vi "Scanner_main_16_3D_2chan.vi"() -> ()   [LabVIEW 2016]
uses:
  <vilib>/DAQmx/write.llb/DAQmx Write (Digital Bool 1Line 1Point).vi
  <vilib>/DAQmx/read.llb/DAQmx Read (Analog 1D DBL 1Chan NSamp).vi
  <vilib>/DAQmx/write.llb/DAQmx Write (Analog 1D Wfm NChan NSamp).vi
  <vilib>/DAQmx/read.llb/DAQmx Read (Counter 1D DBL 1Chan NSamp).vi
  <vilib>/DAQmx/create/channels.llb/DAQmx Create Channel (DO-Digital Output).vi
  <vilib>/DAQmx/miscellaneous.llb/DAQmx Fill In Error Info.vi
  <vilib>/DAQmx/create/channels.llb/DAQmx Create Channel (AI-Voltage-Basic).vi
  <vilib>/DAQmx/configure/timing.llb/DAQmx Timing (Sample Clock).vi
  <vilib>/DAQmx/configure/trigger.llb/DAQmx Start Trigger (Digital Edge).vi
  <vilib>/DAQmx/create/channels.llb/DAQmx Create Channel (CI-Count Edges).vi
  <vilib>/DAQmx/create/channels.llb/DAQmx Create Channel (AO-Voltage-Basic).vi
  <resource>/objmgr/daqmx.rc
panel:
  out "saved .ids":bool
  out "Reflection":dbl[][](graph)
  out "End_of_Stack":bool
  out "refnum out":refnum<file>
  out "Numeric":i32
  out "path to .ids 2":path
  out "x = y?":bool
  out "Z positions":dbl[](array[numeric])
  out "piezo_step":bool
  out "step (um)":dbl
  out "Z position":dbl format="%.6f"
  out "Z step (um)":dbl
  out "System no.":i32=1
  out "Conn. Axes":string[](array[string])
  out "Piezo status":bool
  out "path to .ids":path
  out "saved .ics":bool
  in  "folder":path=path "C:/Users/Sergey/Scan"
  in  "filename":string="PSF2"
  in  "Range Z:":dbl=10.0
  in  "Slices Z:":i32=50
  out "Scan_pix":i32
  out "Frame:":i32
  out "length of scan":i32
  in  "OK Button":bool
  in  "delta_p":i32=-24
  out "Current Line:":i32
  in  "Y":dbl
  in  "offset X:":dbl
  in  "stop":bool
  in  "Save":bool=TRUE
  in  "Range:":dbl=45.0
  in  "Pixels:":i32=650
  in  "Dwell:":dbl=5e-05 format="%#_6p"
  out "Fluorescence":i32[][](graph) caption="Intensity Graph"
  # "Scan:"
  # "Nyquist 0.073um"
  # "Nyquist 0.23um"
  # "Z-position:"
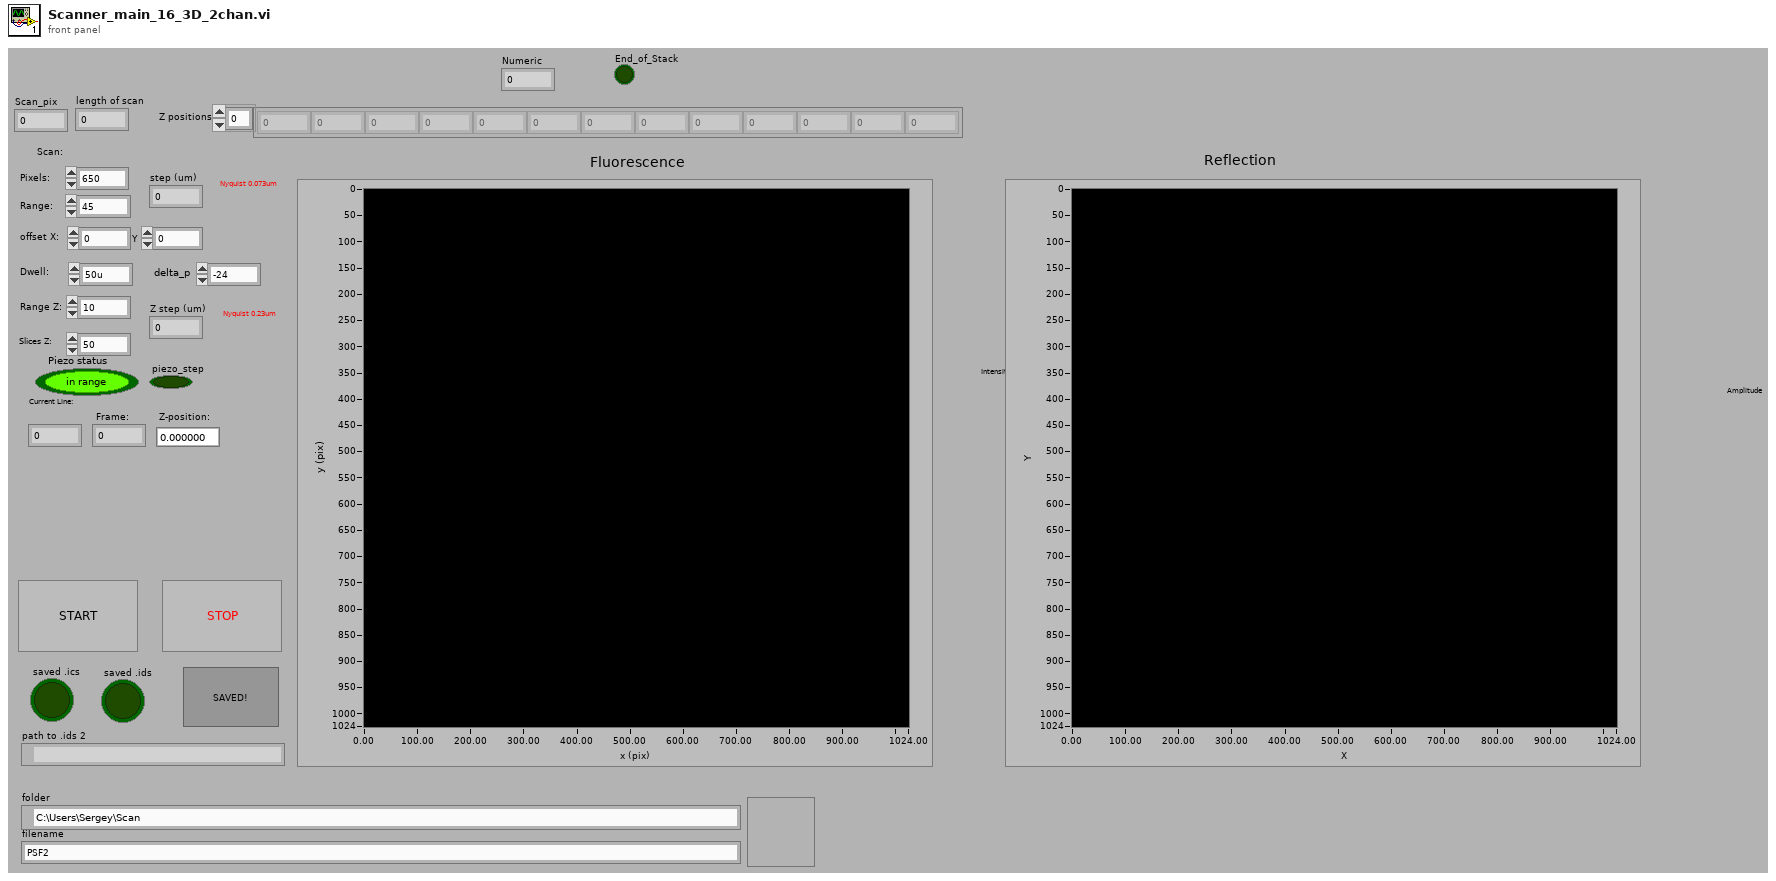
[diagram p1: front panel]
types:
  T1 = enum16{"open", "replace", "create", "open or create", "replace or create", "replace or create with confirmation"}
  T2 = enum16{"big-endian, network order", "native, host order", "little-endian"}
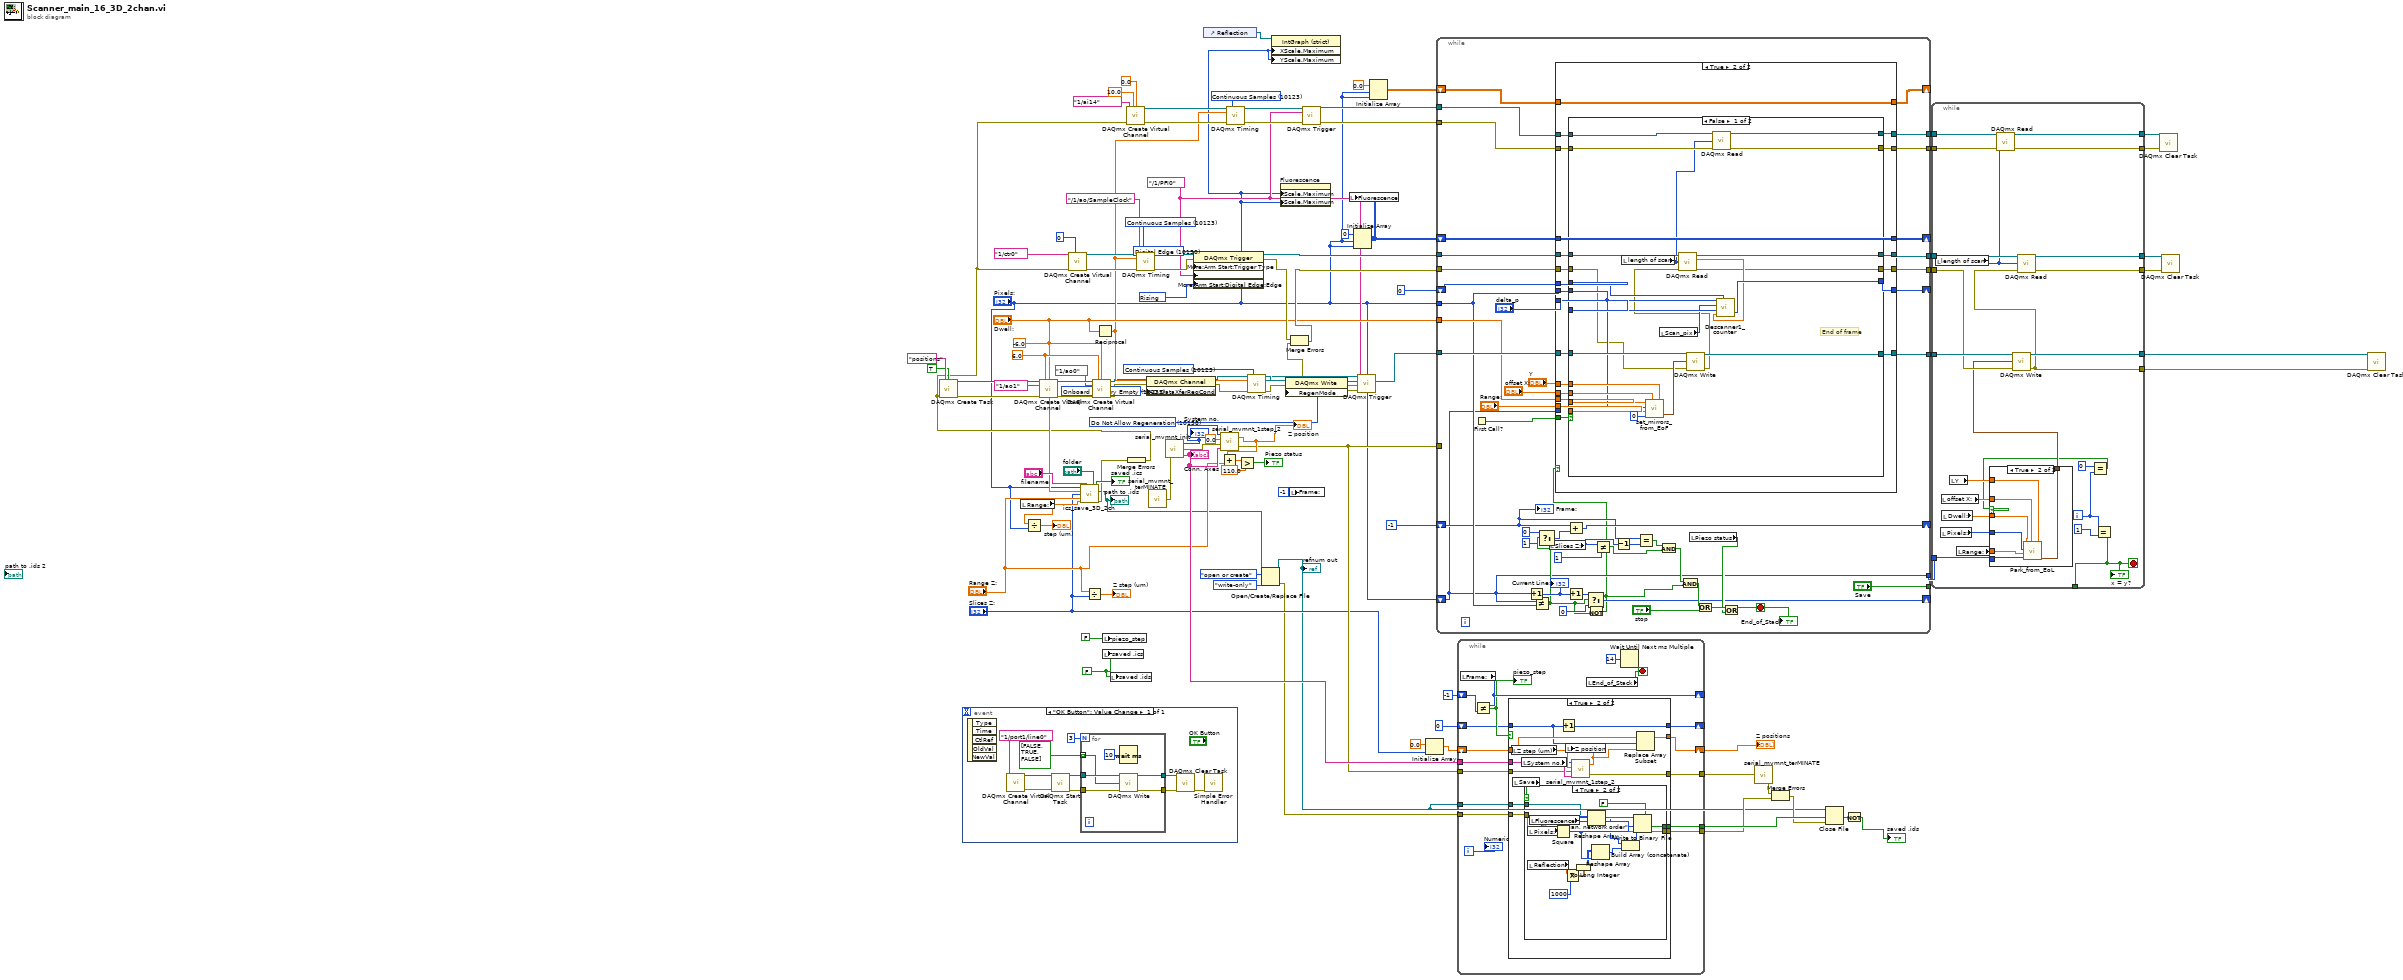
[diagram p0: block diagram]
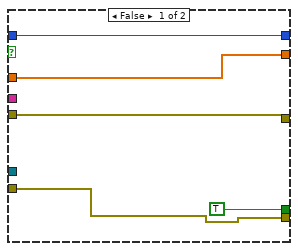
[diagram p2: hidden frame]
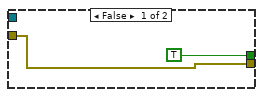
[diagram p3: hidden frame]
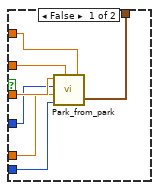
[diagram p4: hidden frame]
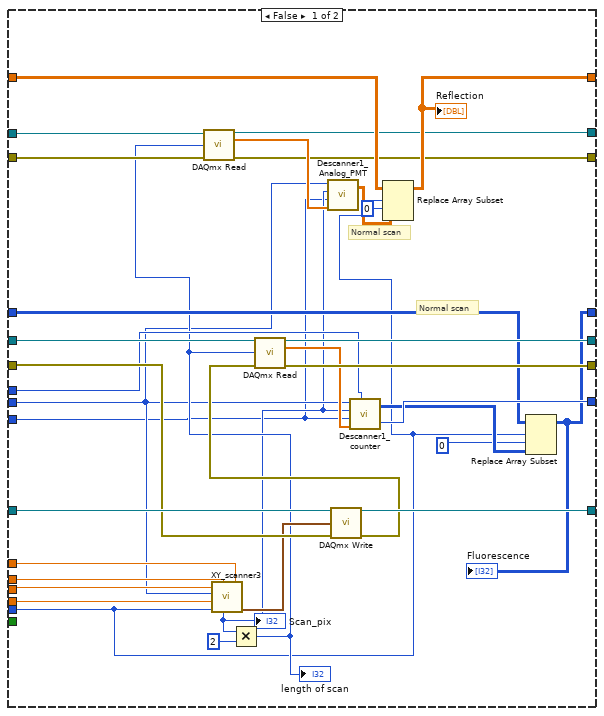
[diagram p5: hidden frame]
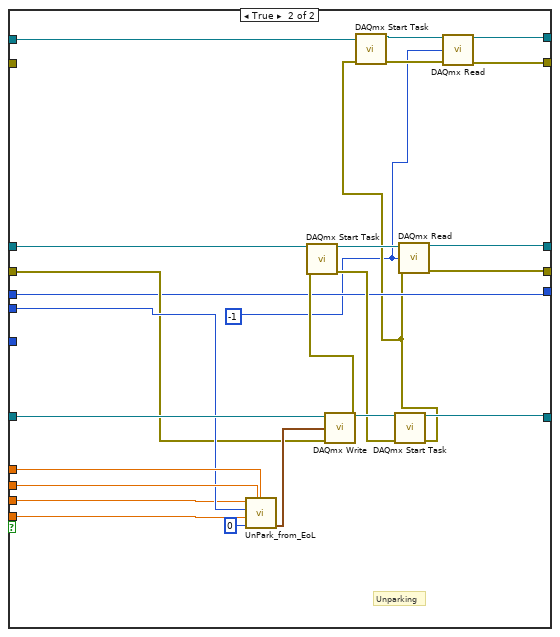
[diagram p6: hidden frame]
diagram:
  w5 = 10235 items=["Onboard Memory Empty"=10235, "Onboard Memory Half Full or Less"=10239, "Onboard Memory Less than Full"=10242] ("AO.DataXferReqCond")
  w30 = 10123 items=["Finite Samples"=10178, "Continuous Samples"=10123] ("sample mode")
  w3 = FALSE ("saved")
  w85 = 10280 items=["Rising"=10280, "Falling"=10171] ("ArmStart.DigEdge.Edge")
  w20 = tag "/1/PFI0" ("ArmStart.DigEdge.Src")
  w86 = 10150 items=["Digital Edge"=10150, "None"=10230] ("ArmStart.TrigType")
  w97 = 10158 items=["Allow Regeneration"=10097, "Do Not Allow Regeneration"=10158] ("RegenMode")
  w101 = 6.0 ("maximum value")
  w100 = -6.0 ("minimum value")
  w105 = 10123 items=["Finite Samples"=10178, "Continuous Samples"=10123] ("sample mode")
  w108 = 10123 items=["Finite Samples"=10178, "Continuous Samples"=10123] ("sample mode")
  n1 = event shown="[0] \"OK Button\": Value Change" {
    selector: _ -> [_]
    dyn-events: _ -> [_]
    timeout: _ -> [_]
    event "OK Button": Value Change {
      n2 = event-data() -> ()  [unwired: 6 out]
      n3 = call-poly <vilib>:"DAQmx Create Virtual Channel.vi"("lines"=tag "1/port1/line0" ("Software Trigger Line")) -> ("task out"=w117:refnum<k21>, "error out"=w116:errorcluster)  [unwired: 4 in, 9 out]
      n4 = call <vilib>:"DAQmx Start Task.vi"("task/channels in"=w117, "error in"=w116) -> ("task out"=w115:refnum<k21>, "error out"=w114:errorcluster)  [unwired: 12 out]
      n5 = for {
        N: 3 -> [_]
        tunnel: w115 -> [w123]
        tunnel: w114 -> [w122]
        tunnel: bool[] [FALSE, TRUE, FALSE] -> [w121] mode=indexing
        tunnel: [w120] -> w111
        tunnel: [w119] -> w110
        n6 = Wait (ms)(milliseconds to wait=u32 10) -> ()  [unwired: 1 out]
        n7 = call-poly <vilib>:"DAQmx Write.vi"("task/channels in"=w123, "data"=w121, "error in"=w122) -> ("task out"=w119:refnum<k21>, "error out"=w120:errorcluster)  [unwired: 1 in, 10 out]
      }
      n8 = call <vilib>:"DAQmx Clear Task.vi"("task in"=w110, "error in"=w111) -> ("error out"=w112:errorcluster)  [unwired: 13 out]
      n9 = call <vilib>:"Simple Error Handler.vi"("error in (no error)"=w112) -> ()  [unwired: 1 in, 8 out]
    }
  }
  n10 = local read "Range:"() -> (w44:dbl)
  n11 = Divide(x=w44, y="Pixels:") -> (x/y=→"step (um)":dbl)
  n12 = call "ics_save_3D_2ch.vi"("pixels"="Pixels:", "filename"="filename", "folder"="folder", "Dwell"="Dwell:", "slices Z"="Slices Z:", "Range Z"="Range Z:", "Range"=w44) -> ("saved"=→"saved .ics":bool, "path to .ids"=w40:path, "error out"=w61:errorcluster)  [unwired: 6 in]
  "path to .ids" <- w40
  n13 = Divide(x="Range Z:", y="Slices Z:") -> (x/y=→"Z step (um)":dbl)
  n14 = Reciprocal(x="Dwell:") -> (1/x=w21:dbl)
  n15 = local write "piezo_step"(FALSE ("x != y?")) -> ()
  n16 = local write "saved .ics"(w3) -> ()
  n17 = local write "saved .ids"(w3) -> ()
  n18 = Merge Errors(w61) -> (w11:errorcluster)
  n19 = call <vilib>:"DAQmx Create Task.vi"("new task name"="positions", "auto cleanup"=TRUE, "error in"=w11) -> ("task out"=w94:refnum<k21>, "error out"=w91:errorcluster)  [unwired: 11 in]
  n20 = call-poly <vilib>:"DAQmx Create Virtual Channel.vi"("task in"=w94, "maximum value"=w101, "minimum value"=w100, "physical channels"=tag "1/ao1", "error in"=w91) -> ("task out"=w104:refnum<k21>, "error out"=w103:errorcluster)  [unwired: 9 in]
  n21 = call-poly <vilib>:"DAQmx Create Virtual Channel.vi"("initial count"=u32 0, "counter"=tag "1/ctr0", "error in"=w11) -> ("task out"=w95:refnum<k21>, "error out"=w107:errorcluster)  [unwired: 11 in]
  n22 = call-poly <vilib>:"DAQmx Create Virtual Channel.vi"("task in"=w104, "maximum value"=w101, "minimum value"=w100, "physical channels"=tag "1/ao0" ("physical channels 2"), "error in"=w103) -> ("task out"=w9:refnum<k21>, "error out"=w7:errorcluster)  [unwired: 9 in]
  n23 = call-poly <vilib>:"DAQmx Create Virtual Channel.vi"("maximum value"=10.0, "minimum value"=0.0, "physical channels"=tag "1/ai14", "error in"=w11) -> ("task out"=w26:refnum<k21>, "error out"=w25:errorcluster)  [unwired: 10 in]
  n24 = call-poly <vilib>:"DAQmx Timing.vi"("task/channels in"=w95, "sample mode"=w108, "rate"=w21, "source"=tag "/1/ao/SampleClock", "error in"=w107) -> ("task out"=w88:refnum<k21>, "error out"=w87:errorcluster)  [unwired: 9 in]
  n25 = property class="DAQmx Channel"(reference=w9, error in=w7, "AO.DataXferReqCond"=w5) -> (reference out=w8:refnum<k21>, error out=w6:errorcluster)
  n26 = call "serial_mvmnt_terMINATE.vi"() -> ("error out"=w55:errorcluster)  [unwired: 1 in]
  n27 = call "serial_mvmnt_init.vi"("error in"=w55) -> ("System no."=w59:i32, "error out"=w58:errorcluster, "Conn. Axes"=w54:string[])
  "Conn. Axes" <- w54
  "System no." <- w59
  n28 = property class="DAQmx Trigger"(reference=w88, error in=w87, "More:Arm Start:Trigger Type"=w86, "More:Arm Start:Digital Edge:Source"=w20, "More:Arm Start:Digital Edge:Edge"=w85) -> (reference out=w79:refnum<k21>, error out=w84:errorcluster)
  n29 = control-ref of="Reflection"() -> (w2:refnum<vi>)
  n30 = call "serial_mvmnt_1step_2.vi"("Conn. Axes"=w54, "error in"=w58, "Z step"=0.0, "System no."=w59) -> ("error out"=w53:errorcluster, "Position"=w56:dbl)
  "Z position" <- w56
  n31 = Add(x=w56, y="Range Z:") -> (x+y=w64:dbl)
  n32 = call-poly <vilib>:"DAQmx Timing.vi"("task/channels in"=w26, "sample mode"=w30, "rate"=w21, "error in"=w25) -> ("task out"=w24:refnum<k21>, "error out"=w23:errorcluster)  [unwired: 10 in]
  n33 = Greater?(x=w64, y=110.0) -> (0:→"Piezo status":bool)
  n34 = call-poly <vilib>:"DAQmx Timing.vi"("task/channels in"=w8, "sample mode"=w105, "rate"=w21, "error in"=w6) -> ("task out"=w99:refnum<k21>, "error out"=w10:errorcluster)  [unwired: 10 in]
  n35 = Open/Create/Replace File(file path (use dialog)=w40, operation (0:open)=T1."open or create", access (0:read/write)=enum16{"read/write", "read-only", "write-only"}."write-only") -> (refnum out=w33:refnum<file>, error out=w38:errorcluster)  [unwired: 3 in, 1 out]
  "refnum out" <- w33
  n36 = property on="Property Node" class="IntGraph (strict)"(reference=w2, "XScale.Maximum"="Pixels:", "YScale.Maximum"="Pixels:") -> ()  [unwired: 1 in, 2 out]
  n37 = property on="Fluorescence" class="IntGraph (strict)"("XScale.Maximum"="Pixels:", "YScale.Maximum"="Pixels:") -> ()  [unwired: 2 in, 2 out]
  n38 = property class="DAQmx Write"(reference=w99, error in=w10, "RegenMode"=w97) -> (reference out=w83:refnum<k21>, error out=w82:errorcluster)
  n39 = local write "Frame:"(-1 ("Frame:")) -> ()
  n40 = call-poly <vilib>:"DAQmx Trigger.vi"("task/channels in"=w24, "source"=w20, "error in"=w23) -> ("task out"=w19:refnum<k21>, "error out"=w18:errorcluster)  [unwired: 11 in]
  n41 = Initialize Array(0 ("element"), "Pixels:", "Pixels:") -> (w37:i32[][])
  n42 = local write "Fluorescence"(w37) -> ()
  n43 = call-poly <vilib>:"DAQmx Trigger.vi"("task/channels in"=w83, "source"=w20, "error in"=w82) -> ("task out"=w80:refnum<k21>, "error out"=w81:errorcluster)  [unwired: 11 in]
  n44 = Merge Errors(w84, w81) -> (w78:errorcluster)
  n45 = Initialize Array(0.0 ("element"), "Pixels:", "Pixels:") -> (w17:dbl[][])
  n46 = Initialize Array(0.0 ("element"), "Slices Z:") -> (w46:dbl[])
  n47 = while {
    tunnel: w80 -> [w162]
    tunnel: w79 -> [w158]
    tunnel: w78 -> [w157]
    tunnel: "Pixels:" -> [w151]
    tunnel: "Dwell:" -> [w153]
    shift-right: [w133] -> _
    shift-left: "Pixels:" -> [w134]
    tunnel: [w165] -> w75
    shift-right: [w159] -> _
    shift-left: w37 -> [w160]
    tunnel: ["Save"] -> _
    tunnel: [w164] -> w76
    tunnel: [w163] -> w77
    tunnel: [w134] -> w71
    shift-right: [w138] -> _
    shift-left: -1 ("t") -> [w135]
    shift-right: [w145] -> _
    shift-left: 0 ("t") -> [w146]
    tunnel: w53 -> [_]
    tunnel: w19 -> [w129]
    tunnel: w18 -> [w128]
    shift-right: [w127] -> _
    shift-left: w17 -> [w130]
    tunnel: [w126] -> w16
    tunnel: [w125] -> w15
    stop <- w131 stop-if-true
    n48 = First Call?() -> (First Call?: T/F=w152:bool)
    n49 = Increment(x=w134) -> (x+1=w168:i32)
    "Current Line:" <- w168
    n50 = Not Equal?(x=w134, y=w151) -> (x != y?=w149:bool)
    n51 = Select(t=0, s=w149, f=1) -> (s? t:f=w150:i32)
    n52 = local read "Slices Z:"() -> (w143:i32)
    n53 = Add(x=w135, y=w150) -> (x+y=w138:i32)
    n54 = Increment(x=w168) -> (x+1=w166:i32)
    n55 = Select(t=w166, s=w149, f=0) -> (s? t:f=w133:i32)
    n56 = Not(x=w149) -> (.not. x?=w132:bool)
    n57 = case shown="True" w132 {
      tunnel: [w202 w225] -> w164
      tunnel: w158 -> [w203 w226]
      tunnel: [w201 w222] -> w165
      tunnel: w157 -> [w194 w221]
      tunnel: [w204 w223] -> w163
      tunnel: w162 -> [w205 w224]
      tunnel: "delta_p" -> [w173 w212]
      tunnel: w151 -> [w175 w215]
      tunnel: w160 -> [w188 w211]
      tunnel: [w186 w211] -> w159
      tunnel: "Y" -> [w200 w220]
      tunnel: "offset X:" -> [w199 w219]
      tunnel: w153 -> [w198 w218]
      tunnel: "Range:" -> [w197 w217]
      tunnel: w134 -> [w172 _]
      tunnel: w152 -> [_ w216]
      tunnel: w146 -> [w192 w213]
      tunnel: [w191 w214] -> w145
      tunnel: w130 -> [w182 w206]
      tunnel: w129 -> [w181 w210]
      tunnel: w128 -> [w180 w209]
      tunnel: [w179 w206] -> w127
      tunnel: [w178 w208] -> w126
      tunnel: [w177 w207] -> w125
      frame False {
        # "Normal scan"
        # "Normal scan"
        n58 = call "XY_scanner3.vi"("offset Y"=w200, "offset X"=w199, "Line_start"=w172, "Range"=w197, "Pixels"=w175, "dwell"=w198) -> ("X and Y"=w193:waveform(dbl)[], "scanPix"=w174:i32)  [unwired: 2 out]
        "Scan_pix" <- w174
        n59 = Multiply(x=w174, y=2) -> (x*y=w176:i32)
        "length of scan" <- w176
        n60 = call-poly <vilib>:"DAQmx Read.vi"("task/channels in"=w181, "number of samples per channel"=w176, "error in"=w180) -> ("task out"=w178:refnum<k21>, "data"=w185:dbl[], "error out"=w177:errorcluster)  [unwired: 10 in]
        n61 = call "Descanner1_Analog_PMT.vi"("Pix"=w175, "scanPix"=w174, "delta_p"=w173, "Data"=w185) -> ("2Lines"=w183:dbl[][])  [unwired: 2 in]
        n62 = call-poly <vilib>:"DAQmx Write.vi"("task/channels in"=w205, "data"=w193, "error in"=w194) -> ("task out"=w204:refnum<k21>, "error out"=w195:errorcluster)  [unwired: 10 in, 1 out]
        n63 = call-poly <vilib>:"DAQmx Read.vi"("task/channels in"=w203, "number of samples per channel"=w176, "error in"=w195) -> ("task out"=w202:refnum<k21>, "data"=w190:dbl[], "error out"=w201:errorcluster)  [unwired: 10 in]
        n64 = call "Descanner1_counter.vi"("Pix"=w175, "scanPix"=w174, "delta_p"=w173, "Data"=w190, "last_count prev line"=w192) -> ("2Lines"=w189:i64[][], "last_count"=w191:i64)
        n65 = Replace Array Subset(array=w182, new element=w183, index (row)=w172, index (col)=0 ("disabled index (col)")) -> (w179:dbl[][])
        "Reflection" <- w179
        n66 = Replace Array Subset(array=w188, new element=w189, index (row)=w172, index (col)=0 ("disabled index (col)")) -> (w186:i32[][])
        "Fluorescence" <- w186
      }
      frame True {
        n67 = case shown="False" w216 {
          tunnel: w226 -> [w250 w264]
          tunnel: [w249 w259] -> w225
          tunnel: w224 -> [w248 w275]
          tunnel: [w247 w266] -> w223
          tunnel: [w232 w258] -> w222
          tunnel: w215 -> [w236 w272]
          tunnel: w221 -> [w233 w265]
          tunnel: w220 -> [w243 w274]
          tunnel: w219 -> [w242 w273]
          tunnel: w218 -> [w245 w271]
          tunnel: w217 -> [w241 w270]
          tunnel: [w239 w261] -> w214
          tunnel: w213 -> [w240 w261]
          tunnel: w212 -> [w237 _]
          tunnel: w210 -> [w231 w251]
          tunnel: w209 -> [w230 _]
          tunnel: [w228 w255] -> w208
          tunnel: [w227 w254] -> w207
          frame False {
            # "End of frame"
            n68 = local read "length of scan"() -> (w229:i32)
            n69 = call "set_mirrors_from_EoF.vi"("offset Y"=w243, "offset X"=w242, "Line_start"=0, "Range"=w241, "Pixels"=w236, "dwell"=w245) -> ("X and Y"=w244:waveform(dbl)[])  [unwired: 1 out]
            n70 = local read "Scan_pix"() -> (w235:i32)
            n71 = call-poly <vilib>:"DAQmx Write.vi"("task/channels in"=w248, "data"=w244, "error in"=w233) -> ("task out"=w247:refnum<k21>, "error out"=w234:errorcluster)  [unwired: 10 in, 1 out]
            n72 = call-poly <vilib>:"DAQmx Read.vi"("task/channels in"=w250, "number of samples per channel"=w229, "error in"=w234) -> ("task out"=w249:refnum<k21>, "data"=w238:dbl[], "error out"=w232:errorcluster)  [unwired: 10 in]
            n73 = call-poly <vilib>:"DAQmx Read.vi"("task/channels in"=w231, "number of samples per channel"=w229, "error in"=w230) -> ("task out"=w228:refnum<k21>, "error out"=w227:errorcluster)  [unwired: 10 in, 1 out]
            n74 = call "Descanner1_counter.vi"("Pix"=w236, "scanPix"=w235, "delta_p"=w237, "Data"=w238, "last_count prev line"=w240) -> ("last_count"=w239:i64)  [unwired: 1 out]
          }
          frame True {
            w252 = -1 ("number of samples per channel")
            # "Unparking"
            n75 = call "UnPark_from_EoL.vi"("offset Y"=w274, "offset X"=w273, "Line_start"=0, "Range"=w270, "Pixels"=w272, "dwell"=w271) -> ("X and Y"=w268:waveform(dbl)[])  [unwired: 2 out]
            n76 = call-poly <vilib>:"DAQmx Write.vi"("task/channels in"=w275, "data"=w268, "error in"=w265) -> ("task out"=w267:refnum<k21>, "error out"=w263:errorcluster)  [unwired: 10 in, 1 out]
            n77 = call <vilib>:"DAQmx Start Task.vi"("task/channels in"=w264, "error in"=w263) -> ("task out"=w260:refnum<k21>, "error out"=w262:errorcluster)  [unwired: 12 in]
            n78 = call <vilib>:"DAQmx Start Task.vi"("task/channels in"=w267, "error in"=w262) -> ("task out"=w266:refnum<k21>, "error out"=w253:errorcluster)  [unwired: 12 in]
            n79 = call <vilib>:"DAQmx Start Task.vi"("task/channels in"=w251, "error in"=w253) -> ("task out"=w257:refnum<k21>, "error out"=w256:errorcluster)  [unwired: 12 in]
            n80 = call-poly <vilib>:"DAQmx Read.vi"("task/channels in"=w260, "number of samples per channel"=w252, "error in"=w253) -> ("task out"=w259:refnum<k21>, "error out"=w258:errorcluster)  [unwired: 10 in, 1 out]
            n81 = call-poly <vilib>:"DAQmx Read.vi"("task/channels in"=w257, "number of samples per channel"=w252, "error in"=w256) -> ("task out"=w255:refnum<k21>, "error out"=w254:errorcluster)  [unwired: 10 in, 1 out]
          }
        }
      }
    }
    n82 = Not Equal?(x=w143, y=1) -> (x != y?=w140:bool)
    n83 = Decrement(x=w143) -> (x-1=w142:i32)
    n84 = Equal?(x=w135, y=w142) -> (x = y?=w141:bool)
    n85 = And(x=w141, y=w140) -> (x .and. y?=w139:bool)
    n86 = And(x=w139, y=w132) -> (x .and. y?=w169:bool)
    n87 = local read "Piezo status"() -> (w136:bool)
    n88 = Or(x=w169, y="stop") -> (x .or. y?=w137:bool)
    n89 = Or(x=w137, y=w136) -> (x .or. y?=w131:bool)
    "End_of_Stack" <- w131
    "Frame:" <- w135
  }
  n90 = while {
    tunnel: w54 -> [w292]
    tunnel: w53 -> [w291]
    shift-right: [w290] -> _
    shift-left: -1 ("Frame") -> [w289]
    tunnel: [w288] -> w51
    shift-right: [w285] -> _
    shift-left: 0 ("Frame") -> [w286]
    shift-right: [w283] -> w32
    shift-left: w46 -> [w284]
    tunnel: [w281] -> w39
    tunnel: w38 -> [w279]
    tunnel: [w278] -> w35
    tunnel: w33 -> [w276]
    i -> [w280]
    stop <- w277 stop-if-true
    n91 = local read "Frame:"() -> (w290:i32)
    n92 = Not Equal?(x=w290, y=w289) -> (x != y?=w287:bool)
    "piezo_step" <- w287
    n93 = case shown="True" w287 {
      tunnel: w292 -> [_ w310]
      tunnel: w291 -> [w297 w309]
      tunnel: [w297 w308] -> w288
      tunnel: w286 -> [w296 w303]
      tunnel: [w296 w304] -> w285
      tunnel: w284 -> [w295 w307]
      tunnel: [w295 w306] -> w283
      tunnel: [TRUE ("cancelled") w301] -> w281
      tunnel: w279 -> [w293 w300]
      tunnel: [w293 w299] -> w278
      tunnel: w276 -> [_ w298]
      frame False {
      }
      frame True {
        n94 = local read "Z step (um)"() -> (w312:dbl)
        n95 = local read "Save"() -> (w302:bool)
        n96 = local read "System no."() -> (w311:i32)
        n97 = case shown="True" w302 {
          tunnel: [TRUE ("cancelled") w327] -> w301
          tunnel: w300 -> [w313 w326]
          tunnel: [w313 w325] -> w299
          tunnel: w298 -> [_ w324]
          frame False {
          }
          frame True {
            n98 = local read "Pixels:"() -> (w329:i32)
            n99 = local read "Reflection"() -> (w322:dbl[][])
            n100 = local read "Fluorescence"() -> (w328:i32[][])
            n101 = Square(x=w329) -> (x^2=w323:i32)
            n102 = Multiply(x=w322, y=1000) -> (x*y=w316:dbl[][])
            n103 = To Long Integer(number=w316) -> (32bit integer=w315:i32[][])
            n104 = Reshape Array(w328, w323) -> (w320:i32[])
            n105 = Reshape Array(w315, w323) -> (w319:i32[])
            n106 = Build Array (concatenate)(w320, w319) -> (w318:i32[])
            n107 = Write to Binary File(file (use dialog)=w324, data=w318, error in=w326, 5:FALSE ("prepend array or string size? (T)"), 9:T2."big-endian, network order" ("byte order (0:big-endian, network order)")) -> (cancelled=w327:bool, error out=w325:errorcluster)  [unwired: 1 in, 1 out]
          }
        }
        n108 = Increment(x=w303) -> (x+1=w304:i32)
        n109 = call "serial_mvmnt_1step_2.vi"("Conn. Axes"=w310, "error in"=w309, "Z step"=w312, "System no."=w311) -> ("error out"=w308:errorcluster, "Position"=w305:dbl)
        n110 = local write "Z position"(w305) -> ()
        n111 = Replace Array Subset(array=w307, new element=w305, index=w303) -> (w306:dbl[])
      }
    }
    n112 = local read "End_of_Stack"() -> (w277:bool)
    n113 = Wait Until Next ms Multiple(millisecond multiple=u32 14 ("milliseconds to wait")) -> ()  [unwired: 1 out]
    "Numeric" <- w280
  }
  "Z positions" <- w32
  n114 = call "serial_mvmnt_terMINATE.vi"("error in"=w51) -> ("error out"=w36:errorcluster)
  n115 = Merge Errors(w36, w35) -> (w34:errorcluster)
  n116 = Close File(refnum=w33, error in=w34) -> ()  [unwired: 2 out]
  n117 = Not(x=w39) -> (.not. x?=→"saved .ids":bool)
  n118 = while {
    tunnel: w77 -> [w354]
    tunnel: w71 -> [w353]
    tunnel: w76 -> [w352]
    tunnel: w75 -> [w351]
    tunnel: [w350] -> w73
    tunnel: [w349] -> w14
    tunnel: [w343] -> w74
    tunnel: [w337] -> w72
    tunnel: [w336] -> _
    tunnel: w16 -> [w335]
    tunnel: w15 -> [w334]
    tunnel: [w332] -> w13
    tunnel: [w331] -> w12
    i -> [w340]
    stop <- w336 stop-if-true
    n119 = local read "length of scan"() -> (w333:i32)
    n120 = local read "Pixels:"() -> (w341:i32)
    n121 = local read "offset X:"() -> (w345:dbl)
    n122 = local read "Dwell:"() -> (w347:dbl)
    n123 = local read "Y"() -> (w346:dbl)
    n124 = local read "Range:"() -> (w348:dbl)
    n125 = call-poly <vilib>:"DAQmx Read.vi"("task/channels in"=w335, "number of samples per channel"=w333, "error in"=w334) -> ("task out"=w332:refnum<k21>, "error out"=w331:errorcluster)  [unwired: 10 in, 1 out]
    n126 = Equal?(x=0, y=w340) -> (x = y?=w338:bool)
    n127 = case shown="True" w338 {
      tunnel: w353 -> [w357 w362]
      tunnel: w348 -> [w358 w363]
      tunnel: w347 -> [w360 w365]
      tunnel: w346 -> [w355 w367]
      tunnel: w345 -> [w356 w366]
      tunnel: [w361 w368] -> w344
      tunnel: w341 -> [w359 w364]
      frame False {
        n128 = call "Park_from_park.vi"("offset Y"=w355, "offset X"=w356, "Line_start"=w357, "Range"=w358, "Pixels"=w359, "dwell"=w360) -> ("X and Y"=w361:waveform(dbl)[])  [unwired: 1 in]
      }
      frame True {
        n129 = call "Park_from_EoL.vi"("offset Y"=w367, "offset X"=w366, "Line_start"=w362, "Range"=w363, "Pixels"=w364, "dwell"=w365) -> ("X and Y"=w368:waveform(dbl)[])  [unwired: 1 in, 2 out]
      }
    }
    n130 = call-poly <vilib>:"DAQmx Write.vi"("task/channels in"=w354, "data"=w344, "error in"=w351) -> ("task out"=w350:refnum<k21>, "error out"=w337:errorcluster)  [unwired: 10 in, 1 out]
    n131 = call-poly <vilib>:"DAQmx Read.vi"("task/channels in"=w352, "number of samples per channel"=w333, "error in"=w337) -> ("task out"=w349:refnum<k21>, "error out"=w343:errorcluster)  [unwired: 10 in, 1 out]
    n132 = Equal?(x=w340, y=1) -> (x = y?=w336:bool)
    "x = y?" <- w336
  }
  n133 = call <vilib>:"DAQmx Clear Task.vi"("task in"=w13, "error in"=w12) -> ()  [unwired: 13 in, 1 out]
  n134 = call <vilib>:"DAQmx Clear Task.vi"("task in"=w14, "error in"=w74) -> ()  [unwired: 13 in, 1 out]
  n135 = call <vilib>:"DAQmx Clear Task.vi"("task in"=w73, "error in"=w72) -> ()  [unwired: 13 in, 1 out]
